vi "Excersize 1.vi"   [LabVIEW 2014, in "Odette_Humirani_5th_LEGORobotics.lvrbt"]
uses:
  Odette_Humirani_5th_LEGORobotics.lvrbt
  <vilib>/NXT/LegoClasses/BrickReference/BrickReference.lvclass
  <vilib>/NXT/Subs/LVHSConnector.ctl
  <vilib>/NXT/NXTIO Xnodes/NXTIOXNode/NXTIO.xnode
  <vilib>/NXT/Hardware/Plugins/Open Port/OpenPortAddress.ctl
  <vilib>/NXT/NXTIO Xnodes/AddressXNode/NXTIOAddress.xnode
  <vilib>/NXT/NXTIO Xnodes/NXTIONodeSubVIs/LEGOMoveAllMotors.vi
types:
  T1 = typedef "OpenPortAddress.ctl" = i32
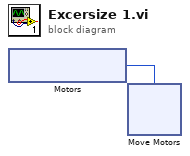
[diagram p0: block diagram]
diagram:
  n1 = xnode "Motors"() -> ("Motor"=w1:T1)
  n2 = xnode "Move Motors"("Motors"=w1) -> ()  [unwired: 2 in, 1 out]
